vi "New.vi"(8 "maximum age [days](None)":dbl=nan, 9 "rollover threshold [MB](50)":dbl=50.0, 10 "formatter (JSON)":refnum<class "Formatter.lvclass">, 11 "log directory (<app dir>/logs)":path) -> (3 "file handler":refnum<class "File Handler.lvclass">)   [LabVIEW 2024, in "Logging.lvlib" / "File Handler.lvclass"]
uses:
  File Handler.lvclass
  Formatters/Formatter/Formatter.lvclass
  File Handler.lvclass/File Handler.ctl
  2cc45319-0579-4416-bf94-d5bc9e63fc92.vi
  Formatters/JSON/JSON.lvclass
  C:/Users/Colin/Documents/LabVIEW/Logging/Formatters/Formatter/Formatter.lvclass
  <vilib>/Utility/LVClass/Get LV Class Name.vi
  <vilib>/Utility/LVClass/Get LV Class Default Value By Name.vi
  Handler/Handler.lvclass
  C:/Users/Colin/Documents/LabVIEW/Logging/Formatters/JSON/JSON.lvclass
  C:/Users/Colin/Documents/LabVIEW/Logging/Handlers/Handler/Handler.lvclass
  C:/Users/Colin/Documents/LabVIEW/Logging/Handlers/File Handler/File Handler.lvclass
panel:
  # "Connector Pane"
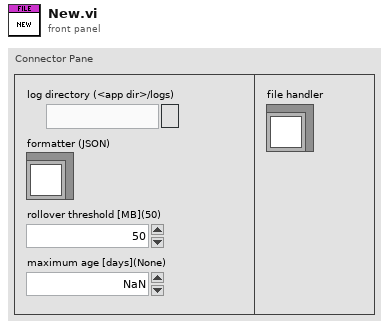
[diagram p1: front panel]
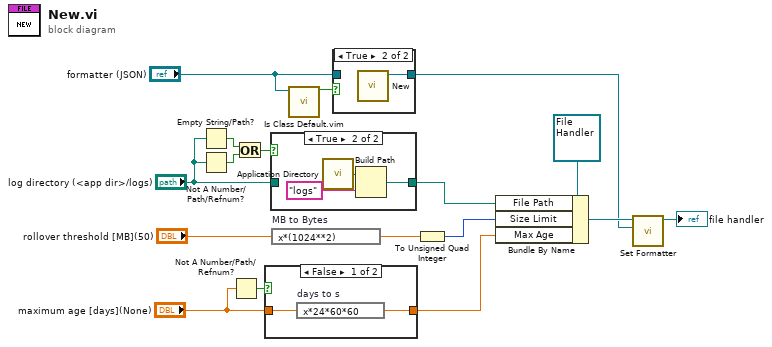
[diagram p0: block diagram]
diagram:
  n1 = Empty String/Path?(string/path="log directory (<app dir>/logs)") -> (empty?=w6:bool)
  n2 = Not A Number/Path/Refnum?(number/path/refnum="log directory (<app dir>/logs)") -> (NaN/Path/Refnum?=w12:bool)
  n3 = Not A Number/Path/Refnum?(number/path/refnum="maximum age [days](None)") -> (NaN/Path/Refnum?=w3:bool)
  n4 = Or(x=w6, y=w12) -> (x .or. y?=w7:bool)
  n5 = case shown="False" w3 {
    tunnel: "maximum age [days](None)" -> [w19 w20]
    tunnel: [w18 w20] -> w13
    frame False {
      n6 = expression code="x*24*60*60" "days to s"(w19) -> (w18:dbl)
    }
    frame True {
    }
  }
  n7 = case shown="True" w7 {
    tunnel: "log directory (<app dir>/logs)" -> [w21 _]
    tunnel: [w21 w22] -> w11
    frame False {
    }
    frame True {
      n8 = call <vilib>:"Application Directory.vi"() -> ("Application Directory"=w24:path)
      n9 = Build Path(base path=w24, name or relative path="logs") -> (appended path=w22:path)
    }
  }
  n10 = expression code="x*(1024**2)" "MB to Bytes"("rollover threshold [MB](50)") -> (w15:dbl)
  n11 = call "Is Class Default.vim"("class"="formatter (JSON)") -> ("is default?"=w10:bool)  [unwired: 9 in, 1 out]
  n12 = case shown="True" w10 {
    tunnel: [w25 w26] -> w1
    tunnel: "formatter (JSON)" -> [w25 _]
    frame False {
    }
    frame True {
      n13 = call "New.vi"() -> ("JSON formatter"=w26:refnum<class "JSON.lvclass">)  [unwired: 11 in]
    }
  }
  n14 = To Unsigned Quad Integer(1:w15) -> (0:w14:u64)
  n15 = Bundle By Name(cluster=refnum<class "File Handler.lvclass"> refnum ("file handler"), "File Path"=w11, "Size Limit"=w14, "Max Age"=w13) -> (w5:refnum<class "File Handler.lvclass">)
  n16 = call "Set Formatter.vi"("formatter"=w1, "handler in"=w5) -> ("handler out"=→"file handler":refnum<class "File Handler.lvclass">)  [unwired: 9 in]
